vi "sqlite3_extended_errcode.vi"(8 "error in (no error)":errorcluster, 11 "psqlite":i64) -> (0 "error out":errorcluster, 3 "extended error code":i32 format="%.0x")   [LabVIEW 2014, in "SQLite3LV.lvlib"]
uses:
  SQLite3LV.lvlib
  sqlite3_64.dll
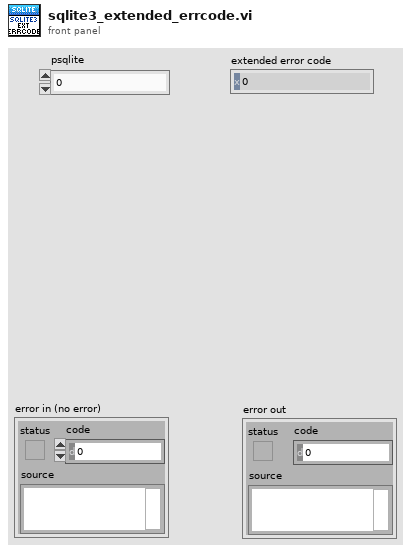
[diagram p1: front panel]
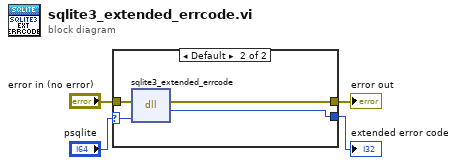
[diagram p0: block diagram]
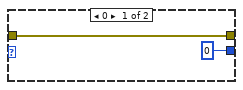
[diagram p2: hidden frame]
diagram:
  n1 = case shown="Default" "psqlite" {
    selector: "psqlite" -> [_ w7]
    tunnel: "error in (no error)" -> [w6 w10]
    tunnel: [w6 w9] -> w3
    tunnel: [0 ("return type") w8] -> w2
    frame 0 {
    }
    frame Default {
      n2 = dll-call lib="C:/Users/BobUser/Desktop/LVTables/sqlite3**.*" fn="sqlite3_extended_errcode"(error in=w10, "psqlite"=w7) -> (error out=w9:errorcluster, "return type"=w8:i32)  [unwired: 3 in, 1 out]
    }
  }
  "error out" <- w3
  "extended error code" <- w2
